vi "iWorx - Circulation Lab.vi"() -> ()   [LabVIEW 2012]
uses:
  <vilib>/DAQmx/read.llb/DAQmx Read (Analog 1D Wfm NChan NSamp).vi
  <vilib>/DAQmx/create/channels.llb/DAQmx Create Channel (AI-Voltage-Basic).vi
  <vilib>/DAQmx/configure/timing.llb/DAQmx Timing (Sample Clock).vi
  <vilib>/measure/macond.llb/IIR Filter for 1 Chan.vi
  <vilib>/DAQmx/miscellaneous.llb/DAQmx Fill In Error Info.vi
  <vilib>/measure/NI_MAPro.lvlib
panel:
  out "Blood Pressure":dbl(knob) scale=-10.0..10.0
  out "Blood Pressure Raw Signal":dbl(knob) scale=-10.0..10.0
  in  "Snapshot BP":bool
  in  "Open Log BP":bool
  in  "Autoscale Y BP":bool
  out "Blood Pressure Chart":waveform(dbl)(graph)
  out "Pulse Chart":waveform(dbl)(graph)
  out "Avg. Pulse":dbl format="%5.1f BPM"
  out "Inst. Pulse":dbl format="%5.1f BPM"
  in  "Threshold":dbl=0.0005 format="%_3p"
  in  "Calibrate":bool
  out "error out":errorcluster
  in  "Set Up":bool
  in  "Pause Button":bool
  in  "Snapshot Pulse":bool
  in  "stop":bool
  in  "Clear Charts":bool caption="Clear Chart"
  in  "Open Log Pulse":bool
  in  "Autoscale Y Pulse":bool
  out "Pulse Raw Signal":dbl(knob) scale=-10.0..10.0
  # "Circulation Lab"
  # "Channel 1"
  # "Channel 2"
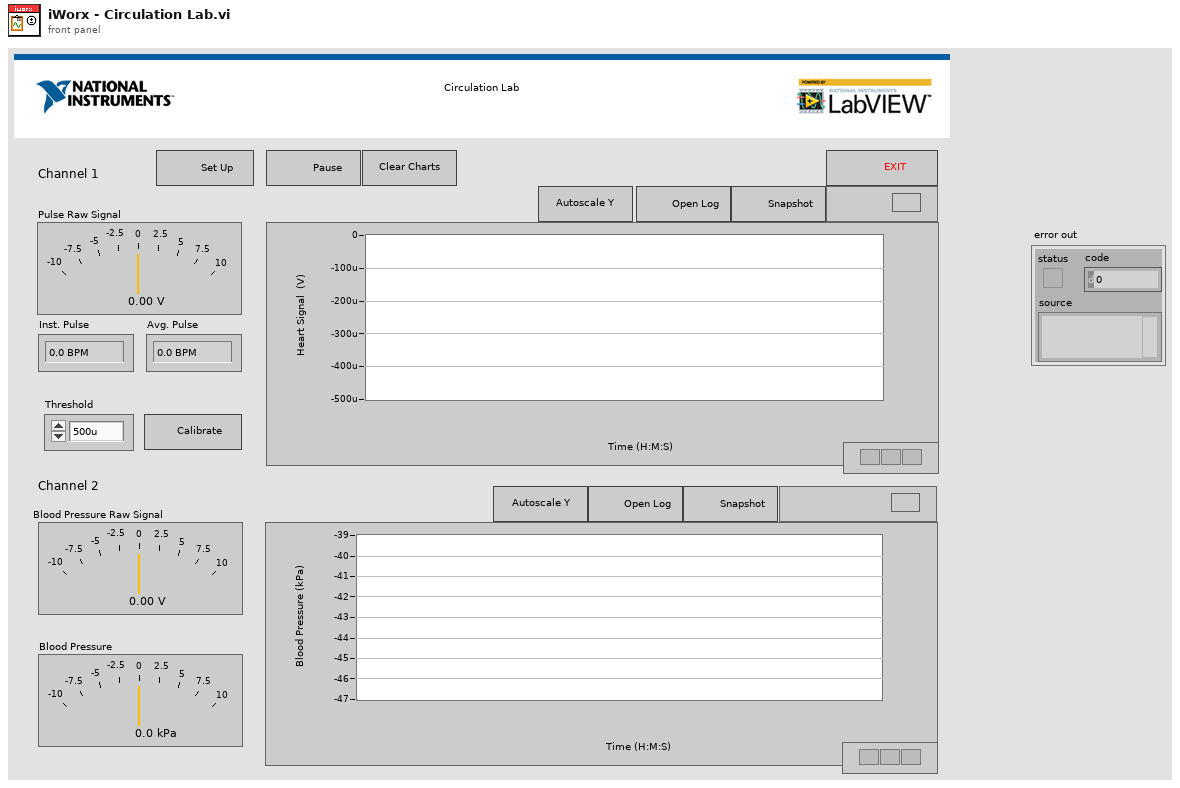
[diagram p1: front panel]
types:
  T1 = cluster{"Topology":enum16{"Off", "Butterworth", "Chebyshev", "Inverse Chebyshev", "Elliptic", "Bessel"}, "Type":enum16{"Lowpass", "Highpass", "Bandpass", "Bandstop"}, "Order":i32, "Lower Fc":dbl, "Upper Fc":dbl, "PB Ripple":dbl, "SB Attenuation":dbl}
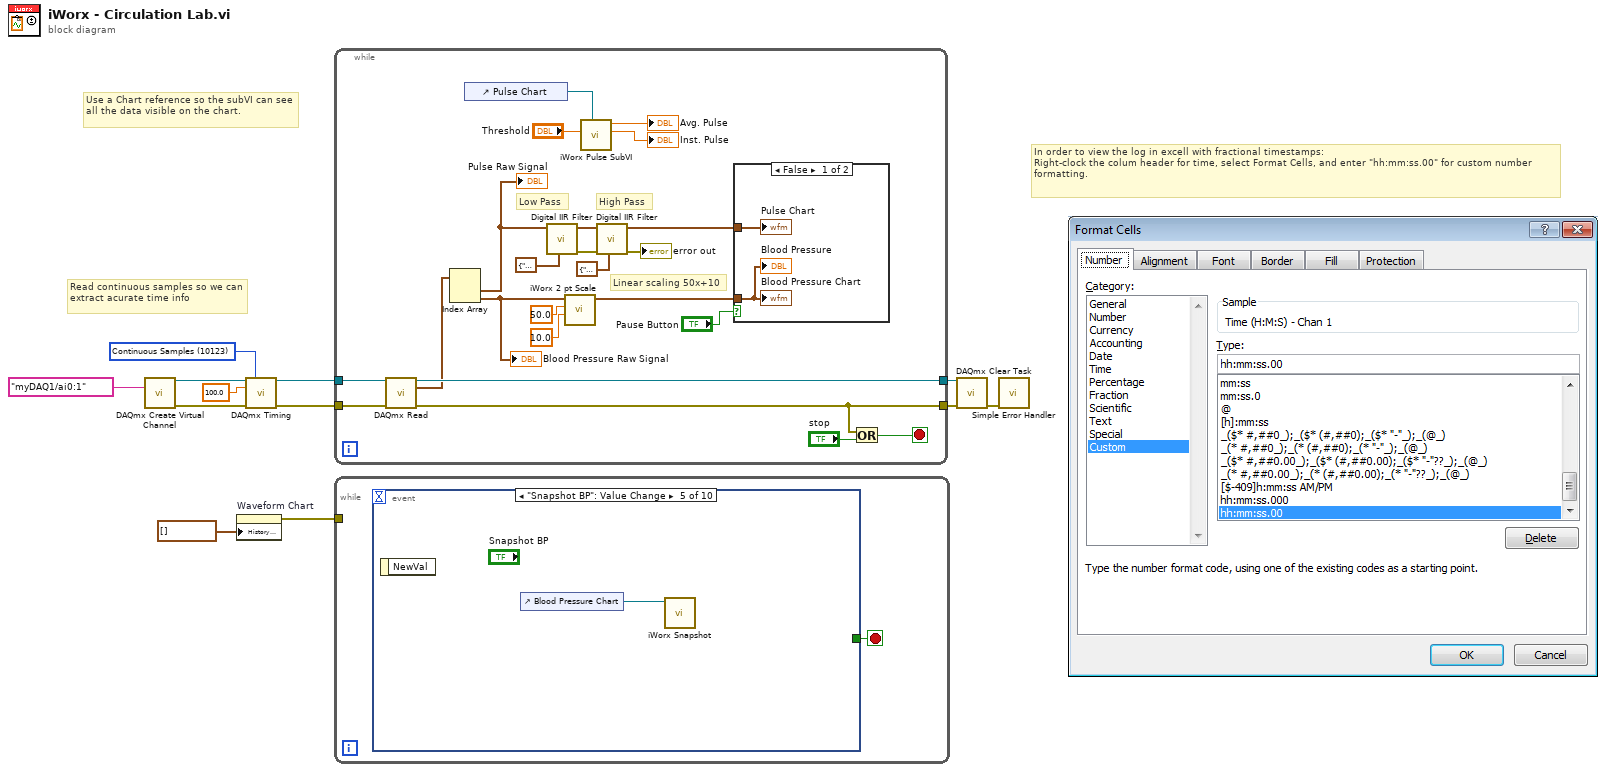
[diagram p0: block diagram]
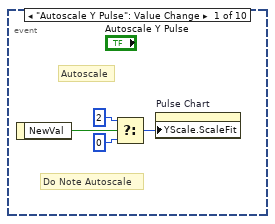
[diagram p2: hidden frame]
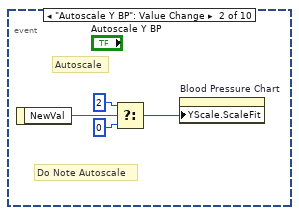
[diagram p3: hidden frame]
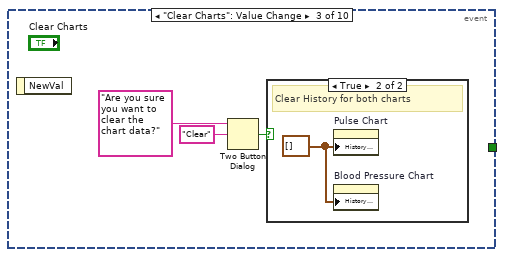
[diagram p4: hidden frame]
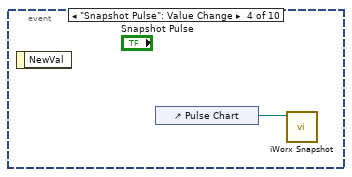
[diagram p6: hidden frame]
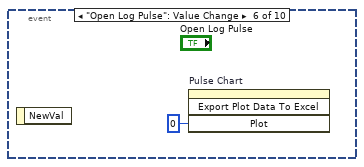
[diagram p7: hidden frame]
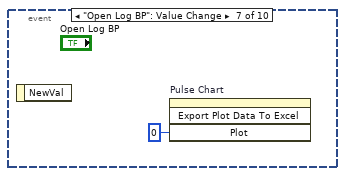
[diagram p8: hidden frame]
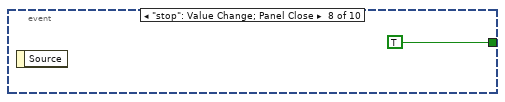
[diagram p9: hidden frame]
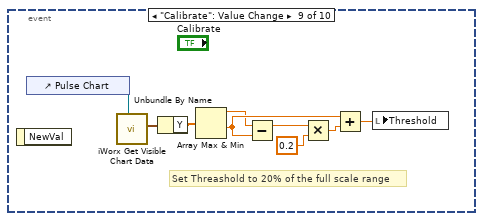
[diagram p10: hidden frame]
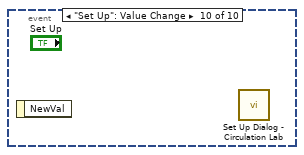
[diagram p11: hidden frame]
diagram:
  w2 = 10123 items=["Finite Samples"=10178, "Continuous Samples"=10123, "Hardware Timed Single Point"=12522] ("sample mode")
  # "Use a Chart reference so the subVI can see all the data visible on the chart."
  # "Read continuous samples so we can extract acurate time info"
  # "In order to view the log in excell with fractional timestamps: \nRight-clock the colum header for time, select Format Cells, and enter \"hh:mm:ss.00\" for custom number formatting."
  n1 = call-poly <vilib>:"DAQmx Create Virtual Channel.vi"("physical channels"=tag "myDAQ1/ai0:1") -> ("task out"=w6:refnum<k21>, "error out"=w5:errorcluster)  [unwired: 13 in]
  n2 = property on="Waveform Chart" class="WFChart (strict)"("History Data"=waveform(dbl)[] []) -> (error out=w7:errorcluster)  [unwired: 2 in, 1 out]
  n3 = call-poly <vilib>:"DAQmx Timing.vi"("task/channels in"=w6, "sample mode"=w2, "rate"=100.0, "error in"=w5) -> ("task out"=w3:refnum<k21>, "error out"=w4:errorcluster)  [unwired: 10 in]
  n4 = while {
    tunnel: w3 -> [w34]
    tunnel: [w33] -> w12
    tunnel: w4 -> [w32]
    tunnel: [w30] -> w11
    stop <- w31 stop-if-true
    # "Linear scaling 50x+10"
    # "High Pass"
    # "Low Pass"
    n5 = call-poly <vilib>:"DAQmx Read.vi"("task/channels in"=w34, "error in"=w32) -> ("task out"=w33:refnum<k21>, "data"=w29:waveform(dbl)[], "error out"=w30:errorcluster)  [unwired: 11 in]
    n6 = Index Array(array=w29) -> (element #1=w22:waveform(dbl), element #2=w18:waveform(dbl))  [unwired: 2 in]
    "Pulse Raw Signal" <- w22
    "Blood Pressure Raw Signal" <- w18
    n7 = control-ref of="Pulse Chart"() -> (w16:refnum<vi>)
    n8 = call-poly <vilib>:"Digital IIR Filter.vi"("IIR filter specifications"=T1 {"Topology"=enum."Butterworth", "Type"=enum."Lowpass", "Order"=1, "Lower Fc"=0.001, "Upper Fc"=200.0, "PB Ripple"=1.0, "SB Attenuation"=60.0}, "signal in"=w22) -> ("error out"=w26:errorcluster, "signal out"=w23:waveform(dbl))  [unwired: 7 in, 1 out]
    n9 = call "iWorx 2 pt Scale.vi"("Offset in"=10.0, "Slope in"=50.0, "Raw Waveform"=w18) -> ("Scaled Value"=w17:waveform(dbl))  [unwired: 6 in, 2 out]
    n10 = call "iWorx Pulse SubVI.vi"("Pulse Chart"=w16, "Threshold (.5mV)"="Threshold") -> ("Inst Pulse Rate (BPM)"=→"Inst. Pulse":dbl, "Average Pulse Rate (BPM)"=→"Avg. Pulse":dbl)  [unwired: 7 in, 1 out]
    n11 = call-poly <vilib>:"Digital IIR Filter.vi"("IIR filter specifications"=T1 {"Topology"=enum."Butterworth", "Type"=enum."Highpass", "Order"=1, "Lower Fc"=1.0, "Upper Fc"=10.0, "PB Ripple"=1.0, "SB Attenuation"=60.0} ("IIR filter specifications 2"), "error in (no error)"=w26, "signal in"=w23) -> ("error out"=→"error out":errorcluster, "signal out"=w25:waveform(dbl))  [unwired: 6 in, 1 out]
    n12 = case shown="False" "Pause Button" {
      tunnel: w25 -> [w37 _]
      tunnel: w17 -> [w36 _]
      frame False {
        "Pulse Chart" <- w37
        "Blood Pressure Chart" <- w36
        "Blood Pressure" <- w36
      }
      frame True {
      }
    }
    n13 = Or(x=w30, y="stop") -> (x .or. y?=w31:bool)
  }
  n14 = while {
    tunnel: w7 -> [_]
    stop <- w38 stop-if-true
    n15 = event shown="[4] \"Snapshot BP\": Value Change" {
      selector: _ -> [_ _ _ _ _ _ _ _ _ _]
      dyn-events: _ -> [_ _ _ _ _ _ _ _ _ _]
      timeout: _ -> [_ _ _ _ _ _ _ _ _ _]
      tunnel: [_ _ _ _ _ _ _ TRUE _ _] -> w38
      event "Autoscale Y Pulse": Value Change {
        # "Do Note Autoscale"
        # "Autoscale"
        n16 = event-data() -> ("NewVal"=w40:bool)  [unwired: 1 in]
        n17 = Select(t=u8 2 ("Y Scale.Scale Fit"), s=w40, f=u8 0 ("Y Scale.Scale Fit")) -> (s? t:f=w39:u8)
        n18 = property on="Pulse Chart" class="WFChart (strict)"("YScale.ScaleFit"=w39) -> ()  [unwired: 2 in, 2 out]
      }
      event "Autoscale Y BP": Value Change {
        # "Do Note Autoscale"
        # "Autoscale"
        n19 = event-data() -> ("NewVal"=w44:bool)  [unwired: 1 in]
        n20 = Select(t=u8 2 ("Y Scale.Scale Fit"), s=w44, f=u8 0 ("Y Scale.Scale Fit")) -> (s? t:f=w43:u8)
        n21 = property on="Blood Pressure Chart" class="WFChart (strict)"("YScale.ScaleFit"=w43) -> ()  [unwired: 2 in, 2 out]
      }
      event "Clear Charts": Value Change {
        n22 = event-data() -> ()  [unwired: 1 in, 1 out]
        n23 = Two Button Dialog(message="Are you sure you want to clear the chart data?", 2:"Clear" ("T button name (\"OK\")")) -> (T button?=w48:bool)  [unwired: 1 in]
        n24 = case shown="True" w48 {
          frame False {
            # "Dialog canceled"
          }
          frame True {
            w50 = waveform(dbl)[] [] ("History Data")
            # "Clear History for both charts"
            n25 = property on="Pulse Chart" class="WFChart (strict)"("History Data"=w50) -> ()  [unwired: 2 in, 2 out]
            n26 = property on="Blood Pressure Chart" class="WFChart (strict)"("History Data"=w50) -> ()  [unwired: 2 in, 2 out]
          }
        }
      }
      event "Snapshot Pulse": Value Change {
        n27 = event-data() -> ()  [unwired: 1 in, 1 out]
        n28 = control-ref of="Pulse Chart"() -> (w51:refnum<vi>)
        n29 = call "iWorx Snapshot.vi"("WaveformChart in"=w51) -> ()  [unwired: 10 in, 1 out]
      }
      event "Snapshot BP": Value Change {
        n30 = event-data() -> ()  [unwired: 1 in, 1 out]
        n31 = control-ref of="Blood Pressure Chart"() -> (w52:refnum<vi>)
        n32 = call "iWorx Snapshot.vi"("WaveformChart in"=w52) -> ()  [unwired: 10 in, 1 out]
      }
      event "Open Log Pulse": Value Change {
        n33 = event-data() -> ()  [unwired: 1 in, 1 out]
        n34 = invoke on="Pulse Chart" class="WFChart (strict)" method="Export Plot Data To Excel"("Plot"=0) -> ()  [unwired: 3 in, 4 out]
      }
      event "Open Log BP": Value Change {
        n35 = event-data() -> ()  [unwired: 1 in, 1 out]
        n36 = invoke on="Pulse Chart" class="WFChart (strict)" method="Export Plot Data To Excel"("Plot"=0) -> ()  [unwired: 3 in, 4 out]
      }
      event "stop": Value Change; Panel Close {
        n37 = event-data() -> ()  [unwired: 1 in, 1 out]
      }
      event "Calibrate": Value Change {
        # "Set Threashold to 20% of the full scale range"
        n38 = event-data() -> ()  [unwired: 1 in, 1 out]
        n39 = control-ref of="Pulse Chart"() -> (w63:refnum<vi>)
        n40 = call "iWorx Get Visible Chart Data.vi"("Selection Chart"=w63) -> ("waveform out"=w64:waveform(dbl))  [unwired: 8 in, 2 out]
        n41 = Unbundle By Name(w64) -> ("Y"=w57:dbl[])
        n42 = Array Max & Min(array=w57) -> (max value=w58:dbl, min value=w62:dbl)  [unwired: 2 out]
        n43 = Subtract(x=w58, y=w62) -> (x-y=w59:dbl)
        n44 = Multiply(x=w59, y=0.2) -> (x*y=w61:dbl)
        n45 = Add(x=w62, y=w61) -> (x+y=w56:dbl)
        n46 = local write "Threshold"(w56) -> ()
      }
      event "Set Up": Value Change {
        n47 = event-data() -> ()  [unwired: 1 in, 1 out]
        n48 = call "Set Up Dialog - Circulation Lab.vi"() -> ()  [unwired: 12 in]
      }
    }
  }
  n49 = call <vilib>:"DAQmx Clear Task.vi"("task in"=w12, "error in"=w11) -> ("error out"=w9:errorcluster)  [unwired: 13 in]
  n50 = call <vilib>:"Simple Error Handler.vi"("error in (no error)"=w9) -> ()  [unwired: 4 in, 5 out]
